vi "set softstart mode.vi"(8 "error in (no error)":errorcluster, 9 "restartdelay":u16, 10 "number":u16, 11 "mode":u16) -> (0 "error out":errorcluster)   [LabVIEW 2015, in "SCANalone4x64.lvlib"]
doc: "__declspec(dllimport) void __stdcall set_softstart_mode(unsigned short mode, unsigned short number, unsigned short restartdelay);"
uses:
  <userlib>/SCANalone4x64/SCANalone4x64.lvlib
  <userlib>/SCANalone4x64/SCANalone4x64.dll
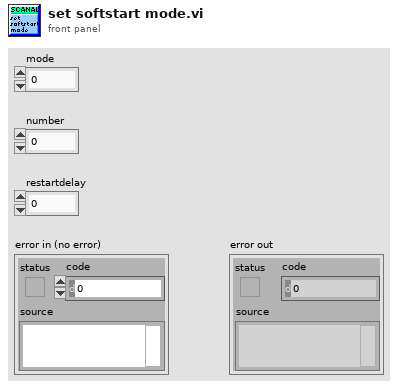
[diagram p1: front panel]
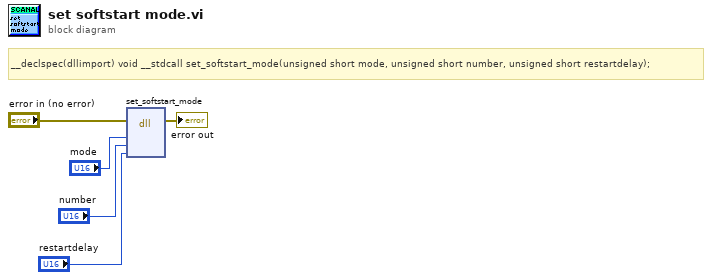
[diagram p0: block diagram]
diagram:
  # "__declspec(dllimport) void __stdcall set_softstart_mode(unsigned short mode, unsigned short number, unsigned short restartdelay);"
  n1 = dll-call lib="C:/Program Files/National Instruments/LabVIEW 2015/user.lib/SCANalone4x64/SCANalone4x64.*" fn="set_softstart_mode"(error in="error in (no error)", "mode"="mode", "number"="number", "restartdelay"="restartdelay") -> (error out=→"error out":errorcluster)  [unwired: 6 in, 1 out]
